vi "Teleop.vi"(10 "Match Info":T1={"Autonomous Elapsed Seconds"=0.0, "TeleOp Elapsed Seconds"=0.0, "Disabled Elapsed Seconds"=0.0, "Visited Autonomous"=FALSE, "Visited TeleOp"=FALSE, "Visited Disabled"=FALSE, "Autonomous Settings"={"Autonomous Style"=enum."Independent", "VI Refnum"=refnum}}, 11 "Call Context":T2) -> ()   [LabVIEW 2011]
doc: "This VI is called for each TeleOp packet received from the DS where the robot is not disabled. It is often used to read from the joysticks and update I/O or to update setpoints for timed control loops. It should complete and return within 20 milliseconds or it may miss DS packets."
uses:
  <vilib>/Rock Robotics/WPI/DriverStation/WPI_DriverStationDerivedRobotMode.ctl
  <vilib>/Rock Robotics/WPI/DriverStation/WPI_DriverStationMatch Info.ctl
  <vilib>/Rock Robotics/WPI/Relay/WPI_RelayValue.ctl
  Robot Global Data.vi
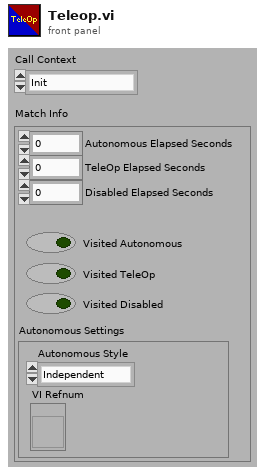
[diagram p1: front panel]
types:
  T1 = typedef "WPI_DriverStationMatch Info.ctl" = cluster{"Autonomous Elapsed Seconds":dbl, "TeleOp Elapsed Seconds":dbl, "Disabled Elapsed Seconds":dbl, "Visited Autonomous":bool, "Visited TeleOp":bool, "Visited Disabled":bool, "Autonomous Settings":cluster{"Autonomous Style":enum16{"Iterative", "Independent"}, "VI Refnum":refnum<vi>}}
  T2 = typedef "WPI_DriverStationDerivedRobotMode.ctl" = enum16{"Init", "Execute", "Stop"}
  T3 = typedef "WPI_RelayValue.ctl" = enum16{"Off", "On", "Forward", "Reverse"}
  T4 = typedef "WPI_JoystickDevRef.ctl" = cluster{"Device":T5}
  T5 = typedef "WPI_JoystickDeviceEnum.ctl" = enum16{"USB 1", "USB 2", "USB 3", "USB 4", "Kinect 1", "Kinect 2"}
  T6 = typedef "WPI_JoystickButtonState.ctl" = cluster{"Button 1":bool, "Button 2":bool, "Button 3":bool, "Button 4":bool, "Button 5":bool, "Button 6":bool, "Button 7":bool, "Button 8":bool, "Button 9":bool, "Button 10":bool, "Button 11":bool, "Button 12":bool}
  T7 = cluster{"axis 1 (x)":dbl, "axis 2 (y)":dbl, "axis 3 (throttle)":dbl, "axis 4":dbl, "axis 5":dbl, "axis 6":dbl}
  T8 = typedef "WPI_MotorControlDeviceRef.ctl" = cluster{"DeviceStatus":errorcluster, "Type":enum16{"PWM", "CAN"}, "PWM":cluster{"Digital Module":T9, "PWM Channel":T10, "DeadBand":T11}, "CAN":cluster{"Device Number":u8, "Control Mode":T12, "Semaphore":T13, "Max Vout":dbl}, "Invert":bool, "TransformRef":T14, "InvTransformRef":T14}
  T9 = typedef "FPGA_TypedefDigitalModule.ctl" = enum16{"Digital Module 1", "Digital Module 2"}
  T10 = typedef "FPGA_DIOPWMChannel.ctl" = enum8{"PWM 1", "PWM 2", "PWM 3", "PWM 4", "PWM 5", "PWM 6", "PWM 7", "PWM 8", "PWM 9", "PWM 10", "Invalid"}
  T11 = typedef "WPI_PWMDeadband.ctl" = cluster{"Name":string, "maxPositivePwm":i32, "minPositivePwm":i32, "centerPwm":i32, "maxNegativePwm":i32, "minNegativePwm":i32, "angularRange":u16}
  T12 = typedef "WPI_CANJaguar_ControlMode.ctl" = enum8{"Percent VBus", "Current", "Speed", "Position", "Voltage"}
  T13 = typedef "Semaphore RefNum" = refnum<k1>
  T14 = typedef "WPI_PWMTransform_ConPane.ctl" = refnum<vi>
  T15 = cluster{"Driver Station Digital Input (1-8)[0]":bool, "Driver Station Digital Input (1-8)[1]":bool, "Driver Station Digital Input (1-8)[2]":bool, "Driver Station Digital Input (1-8)[3]":bool, "Driver Station Digital Input (1-8)[4]":bool, "Driver Station Digital Input (1-8)[5]":bool, "Driver Station Digital Input (1-8)[6]":bool, "Driver Station Digital Input (1-8)[7]":bool, "Driver Station Digital Input (1-8)[8]":bool}
  T16 = typedef "WPI_RelayDevRef.ctl" = cluster{"DevStatus":errorcluster, "Relay Channel":T17, "Digital Module":T9, "Relay Direction":T18}
  T17 = typedef "FPGA_DIORelayChannel.ctl" = enum8{"Relay 1", "Relay 2", "Relay 3", "Relay 4", "Relay 5", "Relay 6", "Relay 7", "Relay 8", "Invalid"}
  T18 = typedef "WPI_RelayDirection.ctl" = enum16{"Both directions", "Forward only", "Reverse only"}
  T19 = typedef "WPI_DigitalInputDevRef.ctl" = cluster{"DevStatus":errorcluster, "DIO Channel":T20, "Digital Module":T9}
  T20 = typedef "FPGA_DIOChannel.ctl" = enum8{"DIO 1", "DIO 2", "DIO 3", "DIO 4", "DIO 5", "DIO 6", "DIO 7", "DIO 8", "DIO 9", "DIO 10", "DIO 11", "DIO 12", "DIO 13", "DIO 14", "Invalid"}
  T21 = typedef "WPI_ServoDeviceRef.ctl" = cluster{"DeviceStatus":errorcluster, "Digital Module":T9, "PWM Channel":T10, "DeadBand":T11}
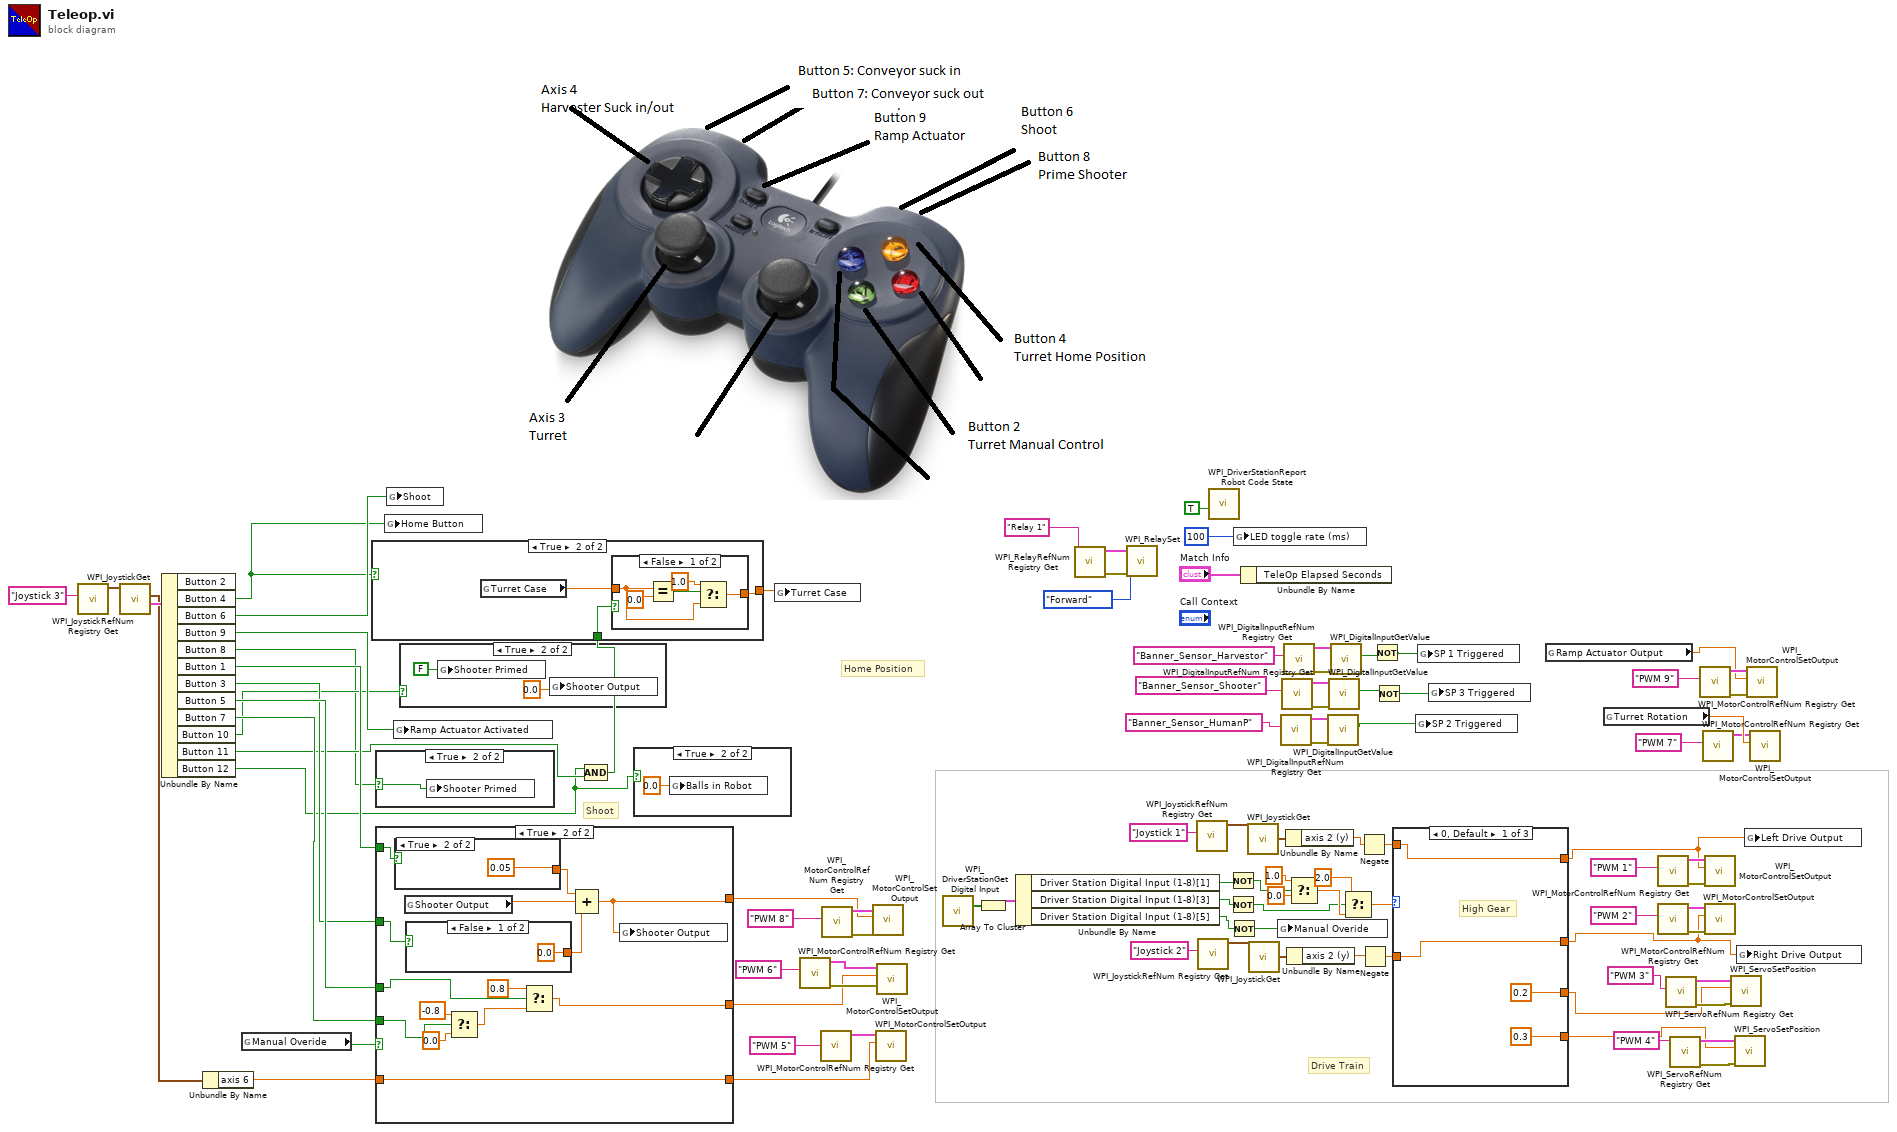
[diagram p0: block diagram]
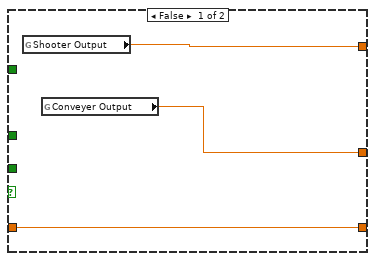
[diagram p4: hidden frame]
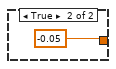
[diagram p5: hidden frame]
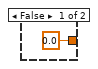
[diagram p6: hidden frame]
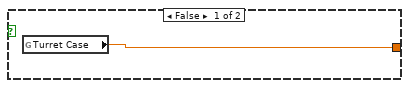
[diagram p8: hidden frame]
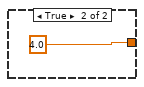
[diagram p9: hidden frame]
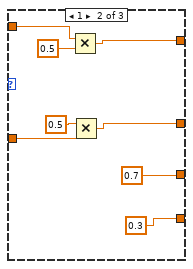
[diagram p10: hidden frame]
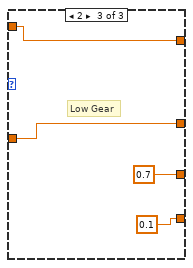
[diagram p11: hidden frame]
diagram:
  # "Shoot"
  # "Home Position"
  # "Drive Train"
  n1 = call <vilib>:"WPI_JoystickRefNum Registry Get.vi"("refnum name"="Joystick 3") -> ("JoystickDevRef"=w49:T4)  [unwired: 9 in, 1 out]
  n2 = call <vilib>:"WPI_JoystickGet.vi"("JoystickDevRef"=w49) -> ("Buttons"=w50:T6, "Axes"=w24:T7)  [unwired: 4 in, 1 out]
  n3 = Unbundle By Name(w50) -> ("Button 4"=w9:bool, "Button 6"=w48:bool, "Button 9"=w52:bool, "Button 8"=w2:bool, "Button 1"=w11:bool, "Button 3"=w10:bool, "Button 5"=w19:bool, "Button 7"=w18:bool, "Button 10"=w3:bool, "Button 11"=w8:bool, "Button 12"=w1:bool)  [unwired: 1 out]
  n4 = Unbundle By Name(w24) -> ("axis 6"=w6:dbl)
  n5 = global read "Robot Global Data.vi" "Manual Overide"() -> (w13:bool)
  n6 = case shown="True" w2 {
    selector: w2 -> [_ w98]
    frame False {
    }
    frame True {
      n7 = global write "Robot Global Data.vi" "Shooter Primed"(w98) -> ()
    }
  }
  n8 = case shown="True" w13 {
    tunnel: [w101 w103] -> w20
    tunnel: w11 -> [_ w108]
    tunnel: w10 -> [_ w107]
    tunnel: w19 -> [_ w110]
    tunnel: w18 -> [_ w111]
    tunnel: [w100 w109] -> w14
    tunnel: [w99 w102] -> w7
    tunnel: w6 -> [w99 w102]
    frame False {
      n9 = global read "Robot Global Data.vi" "Shooter Output"() -> (w101:dbl)
      n10 = global read "Robot Global Data.vi" "Conveyer Output"() -> (w100:dbl)
    }
    frame True {
      n11 = case shown="True" w108 {
        tunnel: [0.0 0.05] -> w106
        frame False {
        }
        frame True {
        }
      }
      n12 = global read "Robot Global Data.vi" "Shooter Output"() -> (w104:dbl)
      n13 = case shown="False" w107 {
        tunnel: [0.0 -0.05] -> w105
        frame False {
        }
        frame True {
        }
      }
      n14 = Select(t=-0.8, s=w111, f=0.0) -> (s? t:f=w115:dbl)
      n15 = Select(t=0.8, s=w110, f=w115) -> (s? t:f=w109:dbl)
      n16 = Compound Arithmetic op=ADD(w106, w104, w105) -> (w103:dbl)
      n17 = global write "Robot Global Data.vi" "Shooter Output"(w103) -> ()
    }
  }
  n18 = global write "Robot Global Data.vi" "Home Button"(w9) -> ()
  n19 = global write "Robot Global Data.vi" "Shoot"(w48) -> ()
  n20 = global write "Robot Global Data.vi" "Ramp Actuator Activated"(w52) -> ()
  n21 = case shown="True" w3 {
    frame False {
    }
    frame True {
      n22 = global write "Robot Global Data.vi" "Shooter Primed"(FALSE ("Shooter Primed")) -> ()
      n23 = global write "Robot Global Data.vi" "Shooter Output"(0.0 ("Shooter Output")) -> ()
    }
  }
  n24 = Compound Arithmetic op=AND(w1, w8) -> (w5:bool)
  n25 = case shown="True" w9 {
    tunnel: [w122 w123] -> w4
    tunnel: w5 -> [_ w125]
    frame False {
      n26 = global read "Robot Global Data.vi" "Turret Case"() -> (w122:dbl)
    }
    frame True {
      n27 = global read "Robot Global Data.vi" "Turret Case"() -> (w124:dbl)
      n28 = case shown="False" w125 {
        tunnel: w124 -> [w127 _]
        tunnel: [w126 4.0 ("Turret Case")] -> w123
        frame False {
          n29 = Equal?(x=w127, y=0.0) -> (x = y?=w129:bool)
          n30 = Select(t=1.0, s=w129, f=w127) -> (s? t:f=w126:dbl)
        }
        frame True {
        }
      }
    }
  }
  n31 = case shown="True" w1 {
    frame False {
    }
    frame True {
      n32 = global write "Robot Global Data.vi" "Balls in Robot"(0.0 ("Balls in Robot")) -> ()
    }
  }
  n33 = global write "Robot Global Data.vi" "Turret Case"(w4) -> ()
  n34 = call <vilib>:"WPI_MotorControlRefNum Registry Get.vi"("refnum name"="PWM 6") -> ("error out"=w15:errorcluster, "MotorControlDevRef"=w16:T8)  [unwired: 9 in]
  n35 = call <vilib>:"WPI_MotorControlRefNum Registry Get.vi"("refnum name"="PWM 5") -> ("MotorControlDevRef"=w42:T8)  [unwired: 9 in, 1 out]
  n36 = call <vilib>:"WPI_MotorControlRefNum Registry Get.vi"("refnum name"="PWM 8") -> ("error out"=w26:errorcluster, "MotorControlDevRef"=w27:T8)  [unwired: 9 in]
  n37 = call <vilib>:"WPI_MotorControlSetOutput.vi"("error in (no error)"=w26, "Output"=w20, "MotorControlDevRef"=w27) -> ()  [unwired: 7 in, 2 out]
  n38 = call <vilib>:"WPI_MotorControlSetOutput.vi"("Output"=w7, "MotorControlDevRef"=w42) -> ()  [unwired: 8 in, 2 out]
  n39 = call <vilib>:"WPI_MotorControlSetOutput.vi"("error in (no error)"=w15, "Output"=w14, "MotorControlDevRef"=w16) -> ()  [unwired: 7 in, 2 out]
  n40 = call <vilib>:"WPI_DriverStationGet Digital Input.vi"() -> ("Driver Station Digital Input (1-8)"=w71:bool[])  [unwired: 11 in]
  n41 = Array To Cluster(array=w71) -> (cluster=w94:T15)
  n42 = Unbundle By Name(w94) -> ("Driver Station Digital Input (1-8)[1]"=w74:bool, "Driver Station Digital Input (1-8)[3]"=w73:bool, "Driver Station Digital Input (1-8)[5]"=w21:bool)
  n43 = call <vilib>:"WPI_RelayRefNum Registry Get.vi"("refnum name"="Relay 1") -> ("error out"=w46:errorcluster, "RelayDevRef"=w47:T16)  [unwired: 9 in]
  n44 = call <vilib>:"WPI_RelaySet.vi"("error in (no error)"=w46, "RelayValue"=WPI_RelayValue."Forward", "RelayDevRef"=w47) -> ()  [unwired: 7 in, 2 out]
  n45 = call <vilib>:"WPI_JoystickRefNum Registry Get.vi"("refnum name"="Joystick 1") -> ("JoystickDevRef"=w87:T4)  [unwired: 9 in, 1 out]
  n46 = call <vilib>:"WPI_JoystickRefNum Registry Get.vi"("refnum name"="Joystick 2") -> ("JoystickDevRef"=w84:T4)  [unwired: 9 in, 1 out]
  n47 = call <vilib>:"WPI_DriverStationReport Robot Code State.vi"("TeleOp"=TRUE ("Autonomous")) -> ()  [unwired: 10 in, 1 out]
  n48 = Not(x=w74) -> (.not. x?=w72:bool)
  n49 = Not(x=w73) -> (.not. x?=w23:bool)
  n50 = Not(x=w21) -> (.not. x?=w22:bool)
  n51 = global write "Robot Global Data.vi" "LED toggle rate (ms)"(u32 100 ("LED ms toggle rate")) -> ()
  n52 = Unbundle By Name("Match Info") -> ()  [unwired: 1 out]
  n53 = call <vilib>:"WPI_JoystickGet.vi"("JoystickDevRef"=w87) -> ("Axes"=w86:T7)  [unwired: 4 in, 2 out]
  n54 = call <vilib>:"WPI_JoystickGet.vi"("JoystickDevRef"=w84) -> ("Axes"=w85:T7)  [unwired: 4 in, 2 out]
  n55 = global write "Robot Global Data.vi" "Manual Overide"(w22) -> ()
  n56 = call <vilib>:"WPI_DigitalInputRefNum Registry Get.vi"("refnum name"="Banner_Sensor_HumanP") -> ("error out"=w37:errorcluster, "DigitalInputDevRef"=w36:T19)  [unwired: 9 in]
  n57 = call <vilib>:"WPI_DigitalInputRefNum Registry Get.vi"("refnum name"="Banner_Sensor_Shooter") -> ("error out"=w38:errorcluster, "DigitalInputDevRef"=w39:T19)  [unwired: 9 in]
  n58 = call <vilib>:"WPI_DigitalInputRefNum Registry Get.vi"("refnum name"="Banner_Sensor_Harvestor") -> ("error out"=w41:errorcluster, "DigitalInputDevRef"=w40:T19)  [unwired: 9 in]
  n59 = Unbundle By Name(w86) -> ("axis 2 (y)"=w70:dbl)
  n60 = Unbundle By Name(w85) -> ("axis 2 (y)"=w68:dbl)
  n61 = Select(t=1.0, s=w72, f=0.0 ("t")) -> (s? t:f=w91:dbl)
  n62 = call <vilib>:"WPI_DigitalInputGetValue.vi"("error in (no error)"=w37, "DigitalInputDevRef"=w36) -> ("Value"=w32:bool)  [unwired: 7 in, 2 out]
  n63 = call <vilib>:"WPI_DigitalInputGetValue.vi"("error in (no error)"=w38, "DigitalInputDevRef"=w39) -> ("Value"=w31:bool)  [unwired: 7 in, 2 out]
  n64 = call <vilib>:"WPI_DigitalInputGetValue.vi"("error in (no error)"=w41, "DigitalInputDevRef"=w40) -> ("Value"=w29:bool)  [unwired: 7 in, 2 out]
  n65 = Select(t=2.0, s=w23, f=w91) -> (s? t:f=w89:dbl)
  n66 = Negate(x=w70) -> (-x=w69:dbl)
  n67 = Negate(x=w68) -> (-x=w67:dbl)
  n68 = Not(x=w29) -> (.not. x?=w28:bool)
  n69 = Not(x=w31) -> (.not. x?=w30:bool)
  n70 = case shown="0, Default" w89 {
    tunnel: w67 -> [w136 w141 w148]
    tunnel: [w136 w142 w148] -> w59
    tunnel: [w135 w143 w147] -> w60
    tunnel: [0.2 ("LeftShifter_Pos") 0.7 0.7] -> w76
    tunnel: [0.3 0.3 ("LeftShifter_Pos") 0.1 ("LeftShifter_Pos")] -> w75
    tunnel: w69 -> [w135 w139 w147]
    frame 0, Default {
      # "High Gear"
    }
    frame 1 {
      n71 = Multiply(x=w139, y=0.5) -> (x*y=w143:dbl)
      n72 = Multiply(x=0.5 ("y"), y=w141) -> (x*y=w142:dbl)
    }
    frame 2 {
      # "Low Gear"
    }
  }
  n73 = global write "Robot Global Data.vi" "SP 2 Triggered"(w32) -> ()
  n74 = global write "Robot Global Data.vi" "SP 1 Triggered"(w28) -> ()
  n75 = global write "Robot Global Data.vi" "SP 3 Triggered"(w30) -> ()
  n76 = global read "Robot Global Data.vi" "Ramp Actuator Output"() -> (w12:dbl)
  n77 = global read "Robot Global Data.vi" "Turret Rotation"() -> (w55:dbl)
  n78 = call <vilib>:"WPI_MotorControlRefNum Registry Get.vi"("refnum name"="PWM 1") -> ("error out"=w64:errorcluster, "MotorControlDevRef"=w66:T8)  [unwired: 9 in]
  n79 = call <vilib>:"WPI_MotorControlRefNum Registry Get.vi"("refnum name"="PWM 2") -> ("error out"=w63:errorcluster, "MotorControlDevRef"=w62:T8)  [unwired: 9 in]
  n80 = call <vilib>:"WPI_ServoRefNum Registry Get.vi"("refnum name"="PWM 3") -> ("error out"=w80:errorcluster, "ServoDeviceRef"=w81:T21)  [unwired: 9 in]
  n81 = call <vilib>:"WPI_ServoRefNum Registry Get.vi"("refnum name"="PWM 4") -> ("error out"=w79:errorcluster, "ServoDeviceRef"=w78:T21)  [unwired: 9 in]
  n82 = call <vilib>:"WPI_MotorControlRefNum Registry Get.vi"("refnum name"="PWM 9") -> ("error out"=w57:errorcluster, "MotorControlDevRef"=w56:T8)  [unwired: 9 in]
  n83 = call <vilib>:"WPI_MotorControlRefNum Registry Get.vi"("refnum name"="PWM 7") -> ("MotorControlDevRef"=w53:T8)  [unwired: 9 in, 1 out]
  n84 = call <vilib>:"WPI_MotorControlSetOutput.vi"("error in (no error)"=w64, "Output"=w60, "MotorControlDevRef"=w66) -> ()  [unwired: 7 in, 2 out]
  n85 = call <vilib>:"WPI_MotorControlSetOutput.vi"("error in (no error)"=w63, "Output"=w59, "MotorControlDevRef"=w62) -> ()  [unwired: 7 in, 2 out]
  n86 = call <vilib>:"WPI_ServoSetPosition.vi"("error in (no error)"=w80, "Position"=w76, "ServoDeviceRef"=w81) -> ()  [unwired: 7 in, 2 out]
  n87 = call <vilib>:"WPI_ServoSetPosition.vi"("error in (no error)"=w79, "Position"=w75, "ServoDeviceRef"=w78) -> ()  [unwired: 7 in, 2 out]
  n88 = global write "Robot Global Data.vi" "Right Drive Output"(w59) -> ()
  n89 = global write "Robot Global Data.vi" "Left Drive Output"(w60) -> ()
  n90 = call <vilib>:"WPI_MotorControlSetOutput.vi"("error in (no error)"=w57, "Output"=w12, "MotorControlDevRef"=w56) -> ()  [unwired: 7 in, 2 out]
  n91 = call <vilib>:"WPI_MotorControlSetOutput.vi"("Output"=w55, "MotorControlDevRef"=w53) -> ()  [unwired: 8 in, 2 out]
